vi "打开文件.vi"(9 "测试人员":string, 11 "错误输入（无错误）":errorcluster) -> (3 "错误输出":errorcluster)   [LabVIEW 2020]
uses:
  <vilib>/drjdpowell/SQLite Library/SQL Connection/Open (path).vi
  <vilib>/drjdpowell/SQLite Library/SQL Connection/Open (string).vi
  <vilib>/AdvancedString/Path To Command Line String.vi
  <vilib>/drjdpowell/SQLite Library/SQL Connection/Execute SQL (No results).vi
  <vilib>/drjdpowell/SQLite Library/SQL Connection/Connection.lvclass
  <vilib>/drjdpowell/SQLite Library/SQLite.lvlib
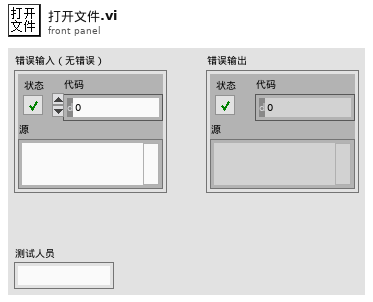
[diagram p1: front panel]
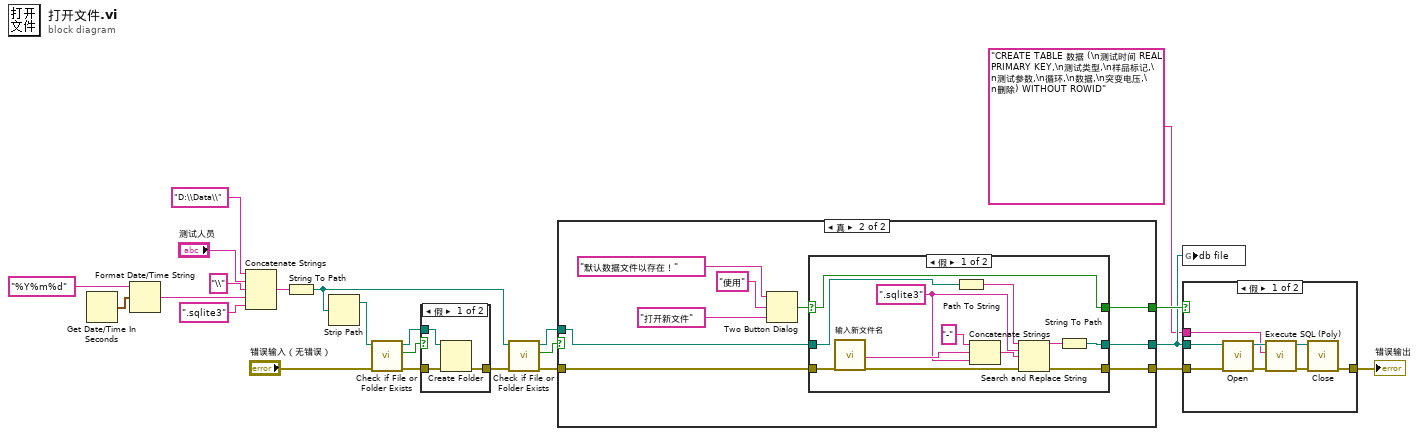
[diagram p0: block diagram]
diagram:
  n1 = Get Date/Time In Seconds() -> (seconds since 1Jan1904=w11:timestamp)
  n2 = Format Date/Time String(time format string (%c)="%Y%m%d" ("时间格式字符串(%c)"), seconds (now)=w11) -> (date/time string=w9:string)  [unwired: 1 in]
  n3 = Concatenate Strings("D:\\Data\\", "测试人员", "\\" ("字符串"), w9, ".sqlite3" ("字符串")) -> (w7:string)
  n4 = String To Path(string=w7) -> (path=w6:path)
  n5 = Strip Path(path=w6) -> (stripped path=w20:path)  [unwired: 1 out]
  n6 = call <vilib>:"Check if File or Folder Exists.vi"("error in (no error)"="错误输入（无错误）", "path"=w20) -> ("error out"=w18:errorcluster, "file or folder exists?"=w17:bool, "dup path"=w19:path)  [unwired: 7 in]
  n7 = case shown="假" w17 {
    tunnel: w19 -> [w26 _]
    tunnel: w18 -> [w25 w27]
    tunnel: [w24 w27] -> w16
    frame False {
      n8 = Create Folder(path (use dialog)=w26, error in=w25) -> (error out=w24:errorcluster)  [unwired: 1 in, 2 out]
    }
    frame True {
    }
  }
  n9 = call <vilib>:"Check if File or Folder Exists.vi"("error in (no error)"=w16, "path"=w6) -> ("error out"=w23:errorcluster, "file or folder exists?"=w22:bool, "dup path"=w21:path)  [unwired: 7 in]
  n10 = case shown="真" w22 {
    selector: w22 -> [w28 _]
    tunnel: w23 -> [w30 w35]
    tunnel: w21 -> [w29 w34]
    tunnel: [w30 w32] -> w5
    tunnel: [w29 w33] -> w2
    tunnel: [w28 w31] -> w3
    frame False {
    }
    frame True {
      n11 = Two Button Dialog(message="默认数据文件以存在！" ("消息"), 1:"打开新文件" ("F按钮名称（“取消”）"), 2:"使用" ("T按钮名称（“确定”）")) -> (T button?=w36:bool)
      n12 = case shown="假" w36 {
        selector: w36 -> [w40 w52]
        tunnel: w35 -> [w45 w53]
        tunnel: w34 -> [w44 w54]
        tunnel: [w42 w54] -> w33
        tunnel: [w41 w53] -> w32
        tunnel: [w40 w52] -> w31
        frame False {
          w46 = ".sqlite3" ("搜索字符串")
          n13 = call "输入新文件名"("error in (no error)"=w45) -> ("输入"=w48:string, "error out"=w50:errorcluster)  [unwired: 16 in, 1 out]
          n14 = Path To String(path=w44) -> (string=w43:string)
          n15 = Concatenate Strings("-" ("字符串"), w48, w46) -> (w49:string)
          n16 = Search and Replace String(input string=w43, search string=w46, replace string=w49, error in=w50) -> (result string=w51:string, error out=w41:errorcluster)  [unwired: 4 in, 2 out]
          n17 = String To Path(string=w51) -> (path=w42:path)
        }
        frame True {
        }
      }
    }
  }
  n18 = global write "数据库.vi" "db file"(w2) -> ()
  n19 = case shown="假" w3 {
    tunnel: w5 -> [w62 w63]
    tunnel: [w57 w63] -> w4
    tunnel: "CREATE TABLE 数据 (\n测试时间 REAL PRIMARY KEY,\n测试类型,\n样品标记,\n测试参数,\n循环,\n数据,\n突变电压,\n删除) WITHOUT ROWID" -> [w58 _]
    tunnel: w2 -> [w55 _]
    frame False {
      n20 = call-poly <vilib>:"Open.vi"("error in (no error)"=w62, "db file"=w55) -> ("error out"=w60:errorcluster, "SQLite Connection"=w61:refnum<class "Connection.lvclass">)  [unwired: 8 in]
      n21 = call-poly <vilib>:"Execute SQL (Poly).vi"("error in (no error)"=w60, "SQL"=w58, "SQLite Connection in"=w61) -> ("error out"=w59:errorcluster, "SQLite Connection"=w56:refnum<class "Connection.lvclass">)  [unwired: 7 in]
      n22 = call-dynamic "Close.vi"("error in (no error)"=w59, "SQLite Connection in"=w56) -> ("error out"=w57:errorcluster)  [unwired: 9 in]
    }
    frame True {
    }
  }
  "错误输出" <- w4
